vi "Validate Name in Section.vi"(8 "error in (no error)":errorcluster, 10 "Name In":string, 11 "Refnum In":T1 format="%.0x") -> (0 "error out":errorcluster, 2 "Name Out":string, 3 "Refnum Out":T1 format="%.0x")   [LabVIEW 2018, in "Instrument Addon Scripting API.lvlib"]
uses:
  Instrument Addon Scripting API.lvlib
  <vilib>/NI Veristand/Custom Device API/Custom Device Item Ref.ctl
  <vilib>/NI Veristand/Custom Device Tools/Custom Device Utility Library/Custom Device Utility Library.lvlib
  <vilib>/NI Veristand/Custom Device API/Custom Device API.lvlib
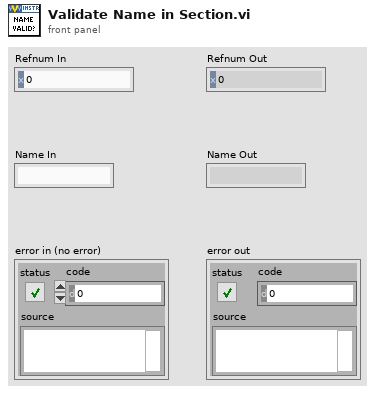
[diagram p1: front panel]
types:
  T1 = typedef "Custom Device API.lvlib/Custom Device Item Ref.ctl" = u64
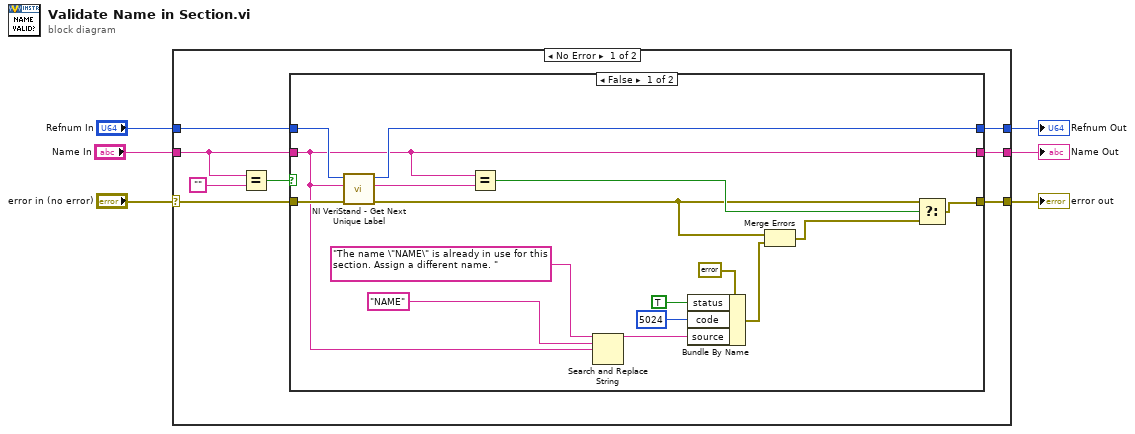
[diagram p0: block diagram]
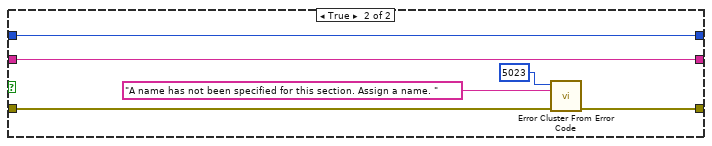
[diagram p2: hidden frame]
diagram:
  n1 = case shown="No Error" "error in (no error)" {
    selector: "error in (no error)" -> [w7 w39]
    tunnel: [w14 w38] -> w6
    tunnel: [w13 w39] -> w5
    tunnel: "Refnum In" -> [w12 w38]
    tunnel: "Name In" -> [w9 w37]
    tunnel: [w8 w37] -> w2
    frame No Error {
      n2 = Equal?(x=w9, y="") -> (x = y?=w10:bool)
      n3 = case shown="False" w10 {
        tunnel: [w30 w36] -> w14
        tunnel: [w25 w34] -> w13
        tunnel: w7 -> [w29 w33]
        tunnel: w12 -> [w28 w36]
        tunnel: w9 -> [w16 w35]
        tunnel: [w16 w35] -> w8
        frame False {
          n4 = call <vilib>:"NI VeriStand - Get Next Unique Label.vi"("error in (no error)"=w29, "Label"=w16, "Parent Ref in"=w28) -> ("error out"=w23:errorcluster, "Label out"=w27:string, "Parent Ref dup"=w30:T1)  [unwired: 5 in, 1 out]
          n5 = Equal?(x=w16, y=w27) -> (x = y?=w26:bool)
          n6 = Search and Replace String(input string="The name \"NAME\" is already in use for this section. Assign a different name. ", search string="NAME", replace string=w16) -> (result string=w21:string)  [unwired: 5 in, 3 out]
          n7 = Bundle By Name(cluster=errorcluster {"status"=FALSE, "code"=0, "source"=""} ("error in (no error)"), "status"=TRUE, "code"=5024, "source"=w21) -> (w15:errorcluster)
          n8 = Merge Errors(w23, w15) -> (w24:errorcluster)
          n9 = Select(t=w23, s=w26, f=w24) -> (s? t:f=w25:errorcluster)
        }
        frame True {
          n10 = call <vilib>:"Error Cluster From Error Code.vi"("error in (no error)"=w33, "error message (\"\")"="A name has not been specified for this section. Assign a name. ", "error code (0)"=5023) -> ("error out"=w34:errorcluster)  [unwired: 6 in]
        }
      }
    }
    frame Error {
    }
  }
  "Refnum Out" <- w6
  "error out" <- w5
  "Name Out" <- w2
